vi "Write Energy.vi"(8 "error in (no error)":errorcluster, 10 "Energy":dbl[unit], 11 "Analyze Parameter Energy in":refnum<class "Analyze Parameter Energy.lvclass">) -> (0 "error out":errorcluster, 3 "Analyze Parameter Energy out":refnum<class "Analyze Parameter Energy.lvclass">)   [LabVIEW 2014, in "Analyze Parameter Energy.lvclass"]
uses:
  Analyze Parameter Energy.lvclass
  Analyze Parameter Energy.lvclass/Analyze Parameter Energy.ctl
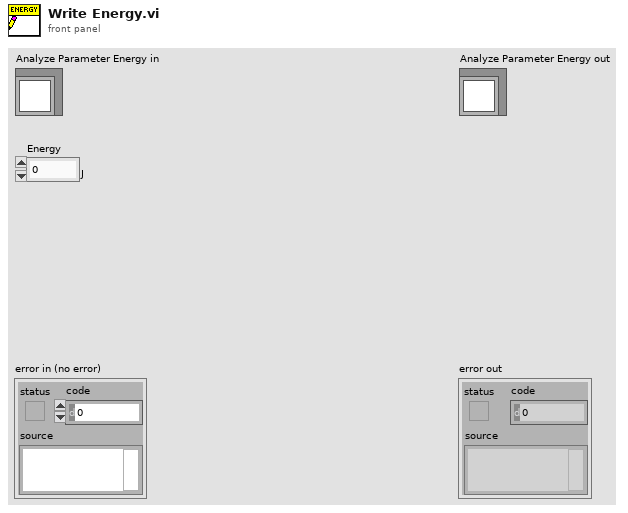
[diagram p1: front panel]
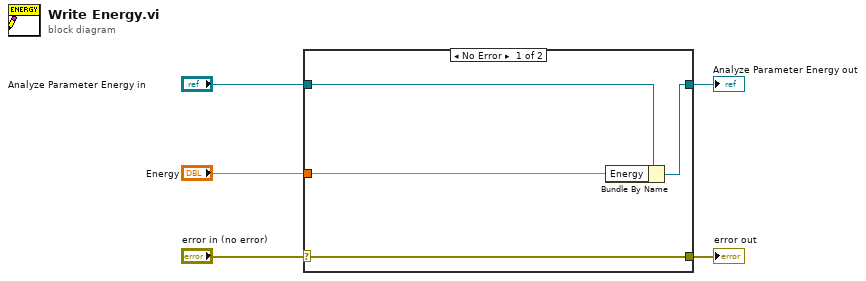
[diagram p0: block diagram]
diagram:
  n1 = case shown="No Error" "error in (no error)" {
    selector: "error in (no error)" -> [w9 w10]
    tunnel: [w9 w10] -> w4
    tunnel: [w7 w11] -> w2
    tunnel: "Analyze Parameter Energy in" -> [w8 w11]
    tunnel: "Energy" -> [w6 _]
    frame No Error {
      n2 = Bundle By Name(cluster=w8, "Energy"=w6) -> (w7:refnum<class "Analyze Parameter Energy.lvclass">)
    }
    frame Error {
    }
  }
  "error out" <- w4
  "Analyze Parameter Energy out" <- w2
